vi "CMD_GET_DPM_CALIBRATION_VALUE.vi"(0 "Input_Data":string[](array[string]), 5 "Error In":errorcluster) -> (12 "Validate CheckSum":bool, 13 "Command":u8[](array[numeric])=[4, 228, 4, 128, 0, 0, 0, 0, 0, 0, 0, 0, 0, 0] format="%x", 14 "Response":bool, 15 "Ack":bool, 16 "Command":bool, 17 "Add CheckSum":bool, 18 "Status":bool, 19 "Error Out":errorcluster)   [LabVIEW 2014]
panel:
  # "Flags"
  # "Get DPM Calibration Command:"
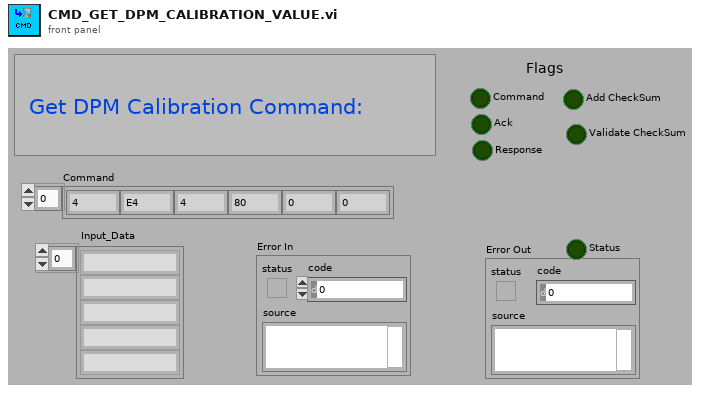
[diagram p1: front panel]
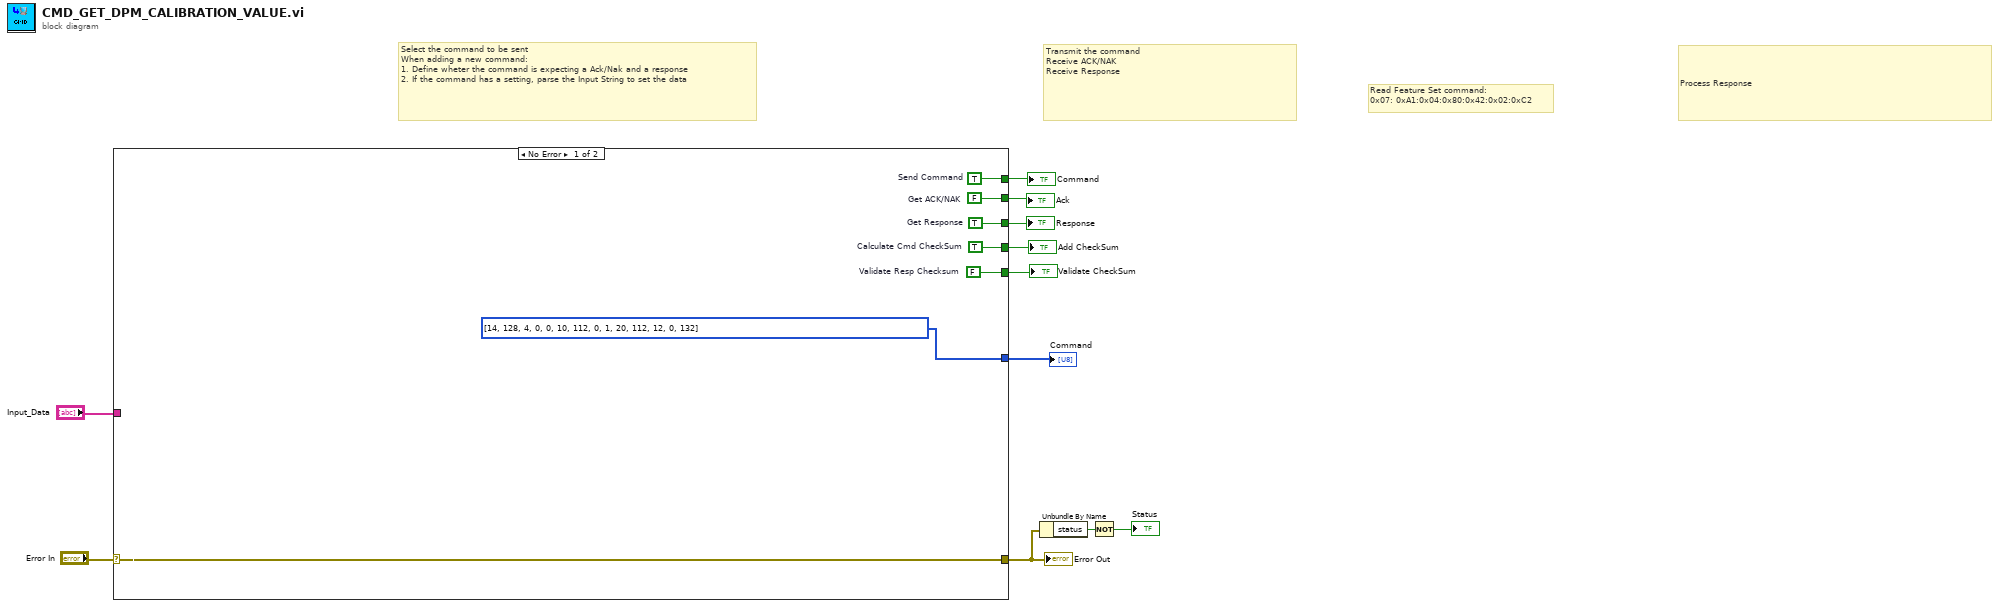
[diagram p0: block diagram]
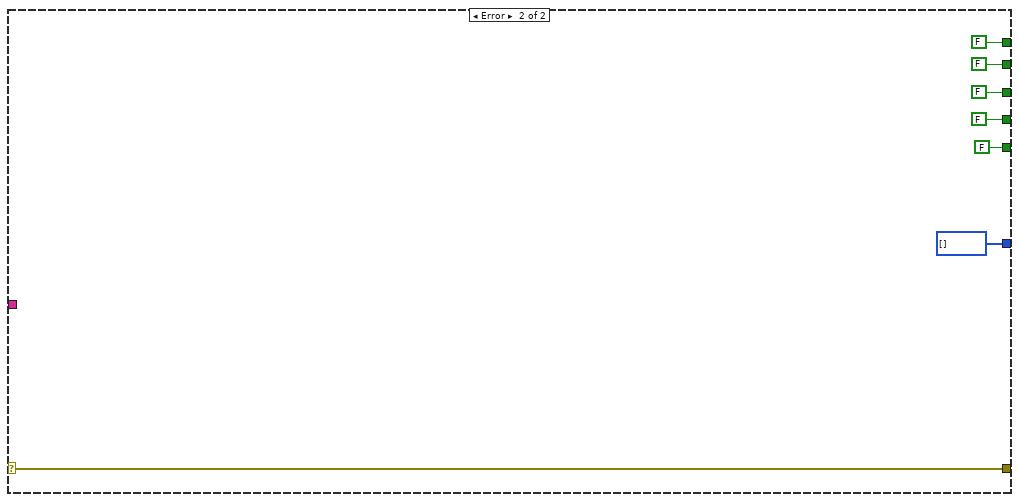
[diagram p2: hidden frame]
diagram:
  # "Read Feature Set command:\n0x07: 0xA1:0x04:0x80:0x42:0x02:0xC2"
  # "Process Response"
  # "Transmit the command\nReceive ACK/NAK\nReceive Response"
  # "Select the command to be sent\nWhen adding a new command:\n1. Define wheter the command is expecting a Ack/Nak and a response\n2. If the command has a setting, parse the Input String to set the data"
  n1 = case shown="No Error" "Error In" {
    selector: "Error In" -> [w14 w20]
    tunnel: [w18 FALSE ("Send Command")] -> w10
    tunnel: [w17 FALSE ("Get ACK/NAK")] -> w9
    tunnel: [w16 FALSE ("Get Response")] -> w8
    tunnel: [w15 FALSE ("Add CheckSum")] -> w7
    tunnel: [u8[] [14, 128, 4, 0, 0, 10, 112, 0, 1, 20, 112, 12, 0, 132] u8[] []] -> w6
    tunnel: [w14 w20] -> w4
    tunnel: "Input_Data" -> [_ _]
    tunnel: [w13 FALSE ("Validate Resp Checksum")] -> w1
    frame No Error {
      w13 = FALSE  # Validate Resp Checksum
      w15 = TRUE  # Calculate Cmd CheckSum
      w16 = TRUE  # Get Response
      w18 = TRUE  # Send Command
      w17 = FALSE  # Get ACK/NAK
    }
    frame Error {
    }
  }
  "Error Out" <- w4
  "Command" <- w10
  "Ack" <- w9
  "Response" <- w8
  "Add CheckSum" <- w7
  "Command" <- w6
  "Validate CheckSum" <- w1
  n2 = Unbundle By Name(w4) -> ("status"=w3:bool)
  n3 = Not(x=w3) -> (.not. x?=→"Status":bool)
